vi "Read Sweep.vi"(8 "error in (no error)":errorcluster, 11 "VISA resource name":refnum<visa-resource-name>) -> (0 "error out":errorcluster, 1 "sweep type":i32(ring) items=["linear sweep", "logarithmic sweep", "frequency list", "CW time sweep", "power sweep"], 3 "VISA resource name out":refnum<visa-resource-name>)   [LabVIEW 2018, in "Agilent 87XX Series.lvlib"]
doc: "This VI for the HP 8753 is used to read the sweep type.\n\n0 LINEAR FREQ\n1 LOG FREQ\n2 LIST FREQ\n3 CW TIME\n4 POWER SWEEP"
uses:
  Agilent 87XX Series.lvlib
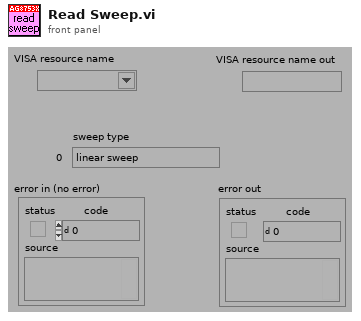
[diagram p1: front panel]
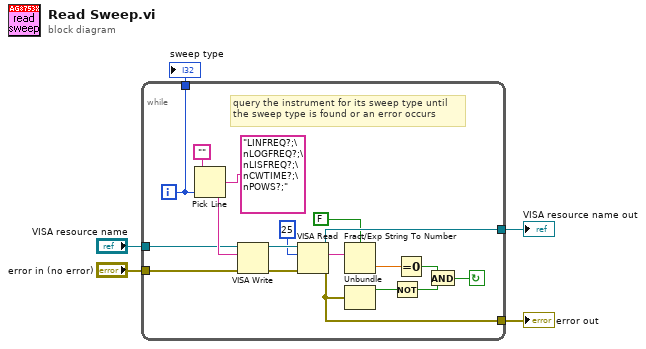
[diagram p0: block diagram]
diagram:
  n1 = while {
    tunnel: [w9] -> w1
    tunnel: [w10] -> w2
    tunnel: "error in (no error)" -> [w11]
    tunnel: "VISA resource name" -> [w12]
    tunnel: [w17] -> w5
    i -> [w17]
    stop <- w13 continue-if-true
    # "query the instrument for its sweep type until\nthe sweep type is found or an error occurs"
    n2 = Pick Line(string ("")="", multi-line string="LINFREQ?;\nLOGFREQ?;\nLISFREQ?;\nCWTIME?;\nPOWS?;", line index=w17) -> (output string=w21:string)
    n3 = VISA Write(VISA resource name=w12, write buffer=w21, error in (no error)=w11) -> (VISA resource name out=w8:refnum<visa-resource-name>, error out=w20:errorcluster)  [unwired: 1 out]
    n4 = VISA Read(VISA resource name=w8, byte count=u32 25, error in (no error)=w20) -> (VISA resource name out=w10:refnum<visa-resource-name>, read buffer=w19:string, error out=w9:errorcluster)  [unwired: 1 out]
    n5 = Fract/Exp String To Number(use system decimal point (T)=FALSE, string=w19) -> (number=w18:dbl)  [unwired: 2 in, 1 out]
    n6 = Unbundle(w9) -> ("status"=w16:bool)  [unwired: 2 out]
    n7 = Not(x=w16) -> (.not. x?=w14:bool)
    n8 = Equal To 0?(x=w18) -> (x = 0?=w15:bool)
    n9 = And(x=w15, y=w14) -> (x .and. y?=w13:bool)
  }
  "sweep type" <- w5
  "VISA resource name out" <- w2
  "error out" <- w1
